vi "BuildErrorCluster.vi"(3 "status type (error:T)":bool=TRUE, 4 "source level (1)":i32=1, 5 "error in (no error)":errorcluster, 6 "ErrorDescription":string, 7 "ErrorCode":i32, 8 "ErrorStatus":bool) -> (0 "error out":errorcluster)   [LabVIEW 2015]
panel:
  # "error\nwarning"
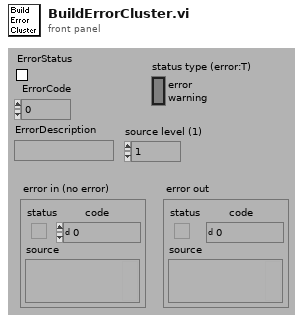
[diagram p1: front panel]
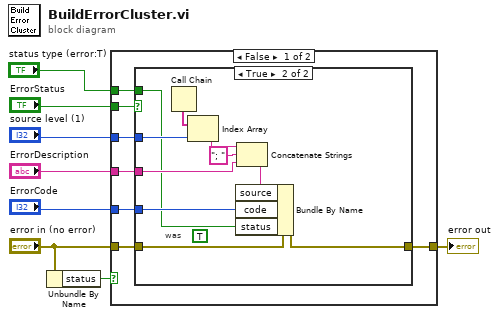
[diagram p0: block diagram]
diagram:
  n1 = Unbundle By Name("error in (no error)") -> ("status"=w8:bool)
  n2 = case shown="False" w8 {
    tunnel: "error in (no error)" -> [w15 w27]
    tunnel: [w13 w27] -> w6
    tunnel: "ErrorCode" -> [w14 _]
    tunnel: "ErrorDescription" -> [w12 _]
    tunnel: "ErrorStatus" -> [w11 _]
    tunnel: "source level (1)" -> [w10 _]
    tunnel: "status type (error:T)" -> [w9 _]
    frame False {
      n3 = case shown="True" w11 {
        tunnel: w15 -> [w16 w26]
        tunnel: w14 -> [_ w25]
        tunnel: [w16 w24] -> w13
        tunnel: w12 -> [_ w19]
        tunnel: w10 -> [_ w22]
        tunnel: w9 -> [_ w17]
        frame False {
        }
        frame True {
          (unwired) TRUE ("status")
          # "was"
          n4 = Call Chain() -> (call chain=w23:string[])
          n5 = Index Array(array=w23, index=w22) -> (element=w21:string)
          n6 = Concatenate Strings(w21, "; ", w19) -> (w18:string)
          n7 = Bundle By Name(cluster=w26, "source"=w18, "code"=w25, "status"=w17) -> (w24:errorcluster)
        }
      }
    }
    frame True {
    }
  }
  "error out" <- w6
